vi "HumanExecute.vi"(8 "error in (no error)":errorcluster) -> (0 "error out":errorcluster)   [LabVIEW 2023]
doc: "Execute for Human\n\ninput:\n error in (cluster)\n\noutput:\n error out (cluster)"
uses:
  <vilib>/Rock Robotics/WPI/Joystick/XBox Axes Indexer.ctl
  <vilib>/Rock Robotics/WPI/Joystick/XBox Buttons Indexer.ctl
  <vilib>/Rock Robotics/WPI/ThirdParty/JAS_Junk/TrajLib/VI/DigSeqLogic_Edge_On.vi
  <vilib>/Rock Robotics/WPI/ThirdParty/JAS_Junk/TrajLib/MathUtil_ApplyDeadband.vi
  Intake/IntakeCancelSendCmd.vi
  Intake/IntakeAlgaeSendCmd.vi
  Intake/IntakeDepositAlgaeSendCmd.vi
  Intake/IntakeCoralSendCmd.vi
  Intake/IntakeDepositCoralSendCmd.vi
  Elevator/ElevatorBargeSendCmd.vi
  Elevator/ElevatorSourceSendCmd.vi
  Elevator/ElevatorFloorSendCmd.vi
  Elevator/ElevSendDecCmd.vi
  Elevator/ElevSendIncCmd.vi
  Elevator/ElevatorCancelCmd.vi
  Elevator/ElevatorL4SendCmd.vi
  Elevator/ElevatorAlgae1SendCmd.vi
  Elevator/ElevatorL3SendCmd.vi
  Elevator/ElevatorAlgae2SendCmd.vi
  Elevator/ElevatorL2SendCmd.vi
  Elevator/ElevatorRestSendCmd.vi
  Elevator/ElevatorL1SendCmd.vi
  HumanGlobal.vi
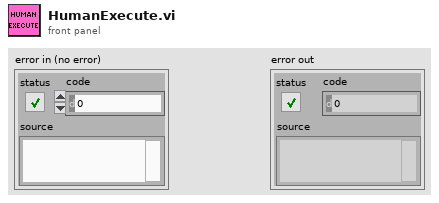
[diagram p1: front panel]
types:
  T1 = typedef "XBox Buttons Indexer.ctl" = enum16{"A", "B", "X", "Y", "Left Bumper", "Right Bumper", "Back", "Start", "Left Joystick", "Right Joystick"}
  T2 = typedef "XBox Axes Indexer.ctl" = enum16{"Left X", "Left Y", "Left Trigger", "Right Trigger", "Right X", "Right Y"}
  T3 = typedef "WPI_JoystickDevRef.ctl" = cluster{"Device":T4}
  T4 = typedef "WPI_JoystickDeviceEnum.ctl" = enum16{"USB 0", "USB 1", "USB 2", "USB 3", "USB 4", "USB 5"}
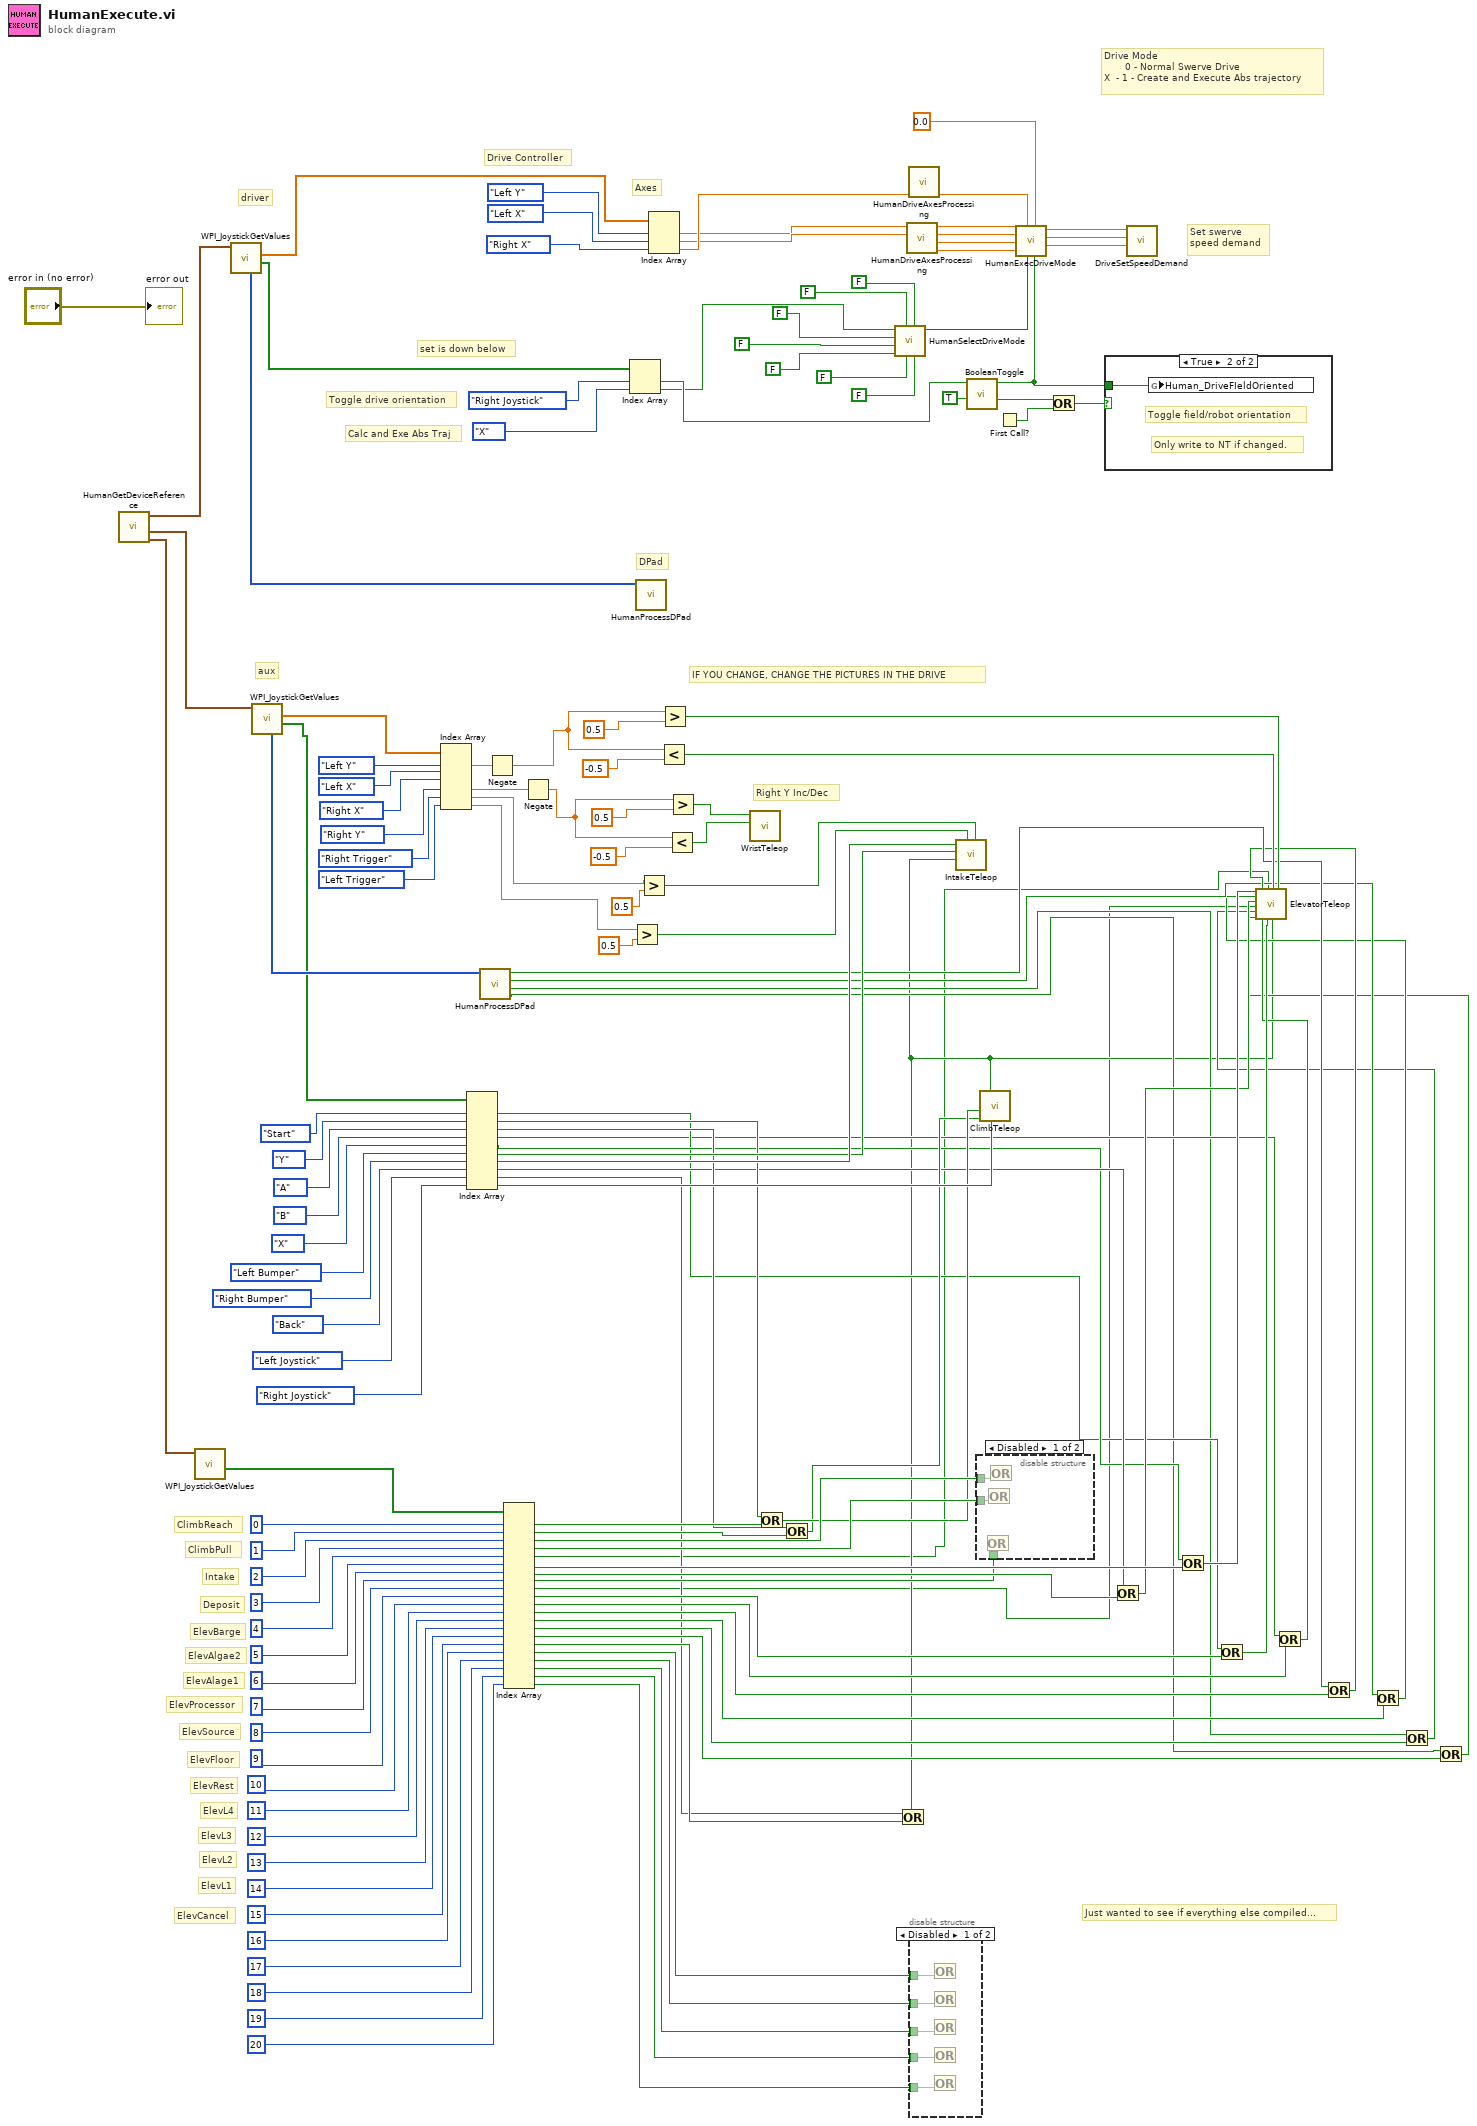
[diagram p0: block diagram]
diagram:
  # "ElevCancel"
  # "ElevL1"
  # "ElevL2"
  # "ElevL3"
  # "ElevL4"
  # "ElevRest"
  # "ElevFloor"
  # "ElevSource"
  # "ElevProcessor"
  # "ElevAlage1"
  # "ElevAlgae2"
  # "ElevBarge"
  # "Deposit"
  # "Intake"
  # "ClimbPull"
  # "ClimbReach"
  # "Just wanted to see if everything else compiled..."
  # "Right Y Inc/Dec"
  # "IF YOU CHANGE, CHANGE THE PICTURES IN THE DRIVE"
  # "DPad"
  # "Toggle drive orientation"
  # "Drive Mode\n       0 - Normal Swerve Drive\nX  - 1 - Create and Execute Abs trajectory"
  # "Calc and Exe Abs Traj"
  # "set is down below"
  # "Set swerve\nspeed demand"
  # "Axes"
  # "Drive Controller"
  # "aux"
  # "driver"
  n1 = call "HumanGetDeviceReference.vi"() -> ("AuxButtonBoard"=w66:T3, "Aux Joy"=w142:T3, "Driver Joy"=w143:T3)  [unwired: 8 in, 1 out]
  n2 = call <vilib>:"WPI_JoystickGetValues.vi"("JoystickDevRef"=w66) -> ("Buttons"=w65:bool[])  [unwired: 6 in, 4 out]
  n3 = call <vilib>:"WPI_JoystickGetValues.vi"("JoystickDevRef"=w143) -> ("Buttons"=w83:bool[], "Axes"=w138:dbl[], "POVs"=w110:i16[])  [unwired: 6 in, 2 out]
  n4 = call <vilib>:"WPI_JoystickGetValues.vi"("JoystickDevRef"=w142) -> ("Buttons"=w112:bool[], "Axes"=w111:dbl[], "POVs"=w113:i16[])  [unwired: 6 in, 2 out]
  n5 = Index Array(array=w111, index #1=XBox_Axes_Indexer."Left Y" ("XBox Axes"), index #2=XBox_Axes_Indexer."Left X" ("XBox Axes"), index #3=XBox_Axes_Indexer."Right X" ("XBox Axes"), index #4=XBox_Axes_Indexer."Right Y" ("XBox Axes"), index #5=XBox_Axes_Indexer."Right Trigger" ("XBox Axes"), index #6=XBox_Axes_Indexer."Left Trigger" ("XBox Axes")) -> (element #1=w70:dbl, element #4=w75:dbl, element #5=w102:dbl, element #6=w101:dbl)  [unwired: 2 out]
  n6 = Index Array "Index Array"(array=w112, index #1=XBox_Buttons_Indexer."Start" ("Nothing"), index #2=XBox_Buttons_Indexer."Y" ("OpenCloseClaw"), index #3=XBox_Buttons_Indexer."A" ("GrabberIn"), index #4=XBox_Buttons_Indexer."B" ("GrabberOut"), index #5=XBox_Buttons_Indexer."X" ("Nothing"), index #6=XBox_Buttons_Indexer."Left Bumper" ("Nothing"), index #7=XBox_Buttons_Indexer."Right Bumper" ("Nothing"), index #8=XBox_Buttons_Indexer."Back" ("Place Cone"), index #9=XBox_Buttons_Indexer."Left Joystick" ("Place Cone"), index #10=XBox_Buttons_Indexer."Right Joystick" ("Place Cone")) -> (element #1=w16:bool, element #2=w25:bool, element #3=w23:bool, element #4=w14:bool, element #5=w17:bool, element #6=w80:bool, element #7=w98:bool, element #8=w20:bool, element #9=w4:bool, element #10=w73:bool)
  n7 = call "HumanProcessDPad.vi"("POV"=w113) -> ("Left"=w6:bool, "Down"=w8:bool, "Right"=w10:bool, "Up"=w12:bool)  [unwired: 7 in]
  n8 = Negate(x=w70) -> (-x=w69:dbl)
  n9 = Index Array "Index Array"(array=w65, index #1=0 ("index"), index #2=1 ("index"), index #3=2 ("index"), index #4=3 ("index"), index #5=4 ("index"), index #6=5 ("index"), index #7=6 ("index"), index #8=7 ("index"), index #9=8 ("index"), index #10=9 ("index"), index #11=10 ("index"), index #12=11 ("index"), index #13=12 ("index"), index #14=13 ("index"), index #15=14 ("index"), index #16=15 ("index"), index #17=16 ("index"), index #18=17 ("index"), index #19=18 ("index"), index #20=19 ("index"), index #21=20 ("index")) -> (element #1=w43:bool, element #2=w42:bool, element #3=w41:bool, element #4=w40:bool, element #5=w2:bool, element #6=w39:bool, element #7=w38:bool, element #8=w18:bool, element #9=w1:bool, element #10=w37:bool, element #11=w36:bool, element #12=w35:bool, element #13=w34:bool, element #14=w33:bool, element #15=w32:bool, element #16=w31:bool, element #17=w30:bool, element #18=w29:bool, element #19=w28:bool, element #20=w27:bool, element #21=w26:bool)
  n10 = Negate(x=w75) -> (-x=w74:dbl)
  n11 = Index Array(array=w83, index #1=XBox_Buttons_Indexer."Right Joystick" ("Nothing"), index #2=XBox_Buttons_Indexer."X" ("Nothing")) -> (element #1=w81:bool, element #2=w77:bool)
  n12 = Greater?(x=w101, y=0.5) -> (0:w99:bool)
  n13 = call "HumanProcessDPad.vi"("POV"=w110) -> ()  [unwired: 7 in, 4 out]
  n14 = Greater?(x=w102, y=0.5) -> (0:w100:bool)
  n15 = Index Array(array=w138, index #1=XBox_Axes_Indexer."Left Y" ("XBox Axes"), index #2=XBox_Axes_Indexer."Left X" ("XBox Axes"), index #3=XBox_Axes_Indexer."Right X" ("XBox Axes")) -> (element #1=w127:dbl, element #2=w128:dbl, element #3=w129:dbl)
  n16 = Less?(x=w69, y=-0.5) -> (x < y?=w71:bool)
  n17 = Greater?(x=w69, y=0.5) -> (0:w72:bool)
  n18 = Less?(x=w74, y=-0.5) -> (x < y?=w67:bool)
  n19 = Greater?(x=w74, y=0.5) -> (0:w68:bool)
  n20 = call "WristTeleop.vi"("Dec"=w67, "Inc"=w68) -> ()  [unwired: 10 in]
  n21 = Or(x=w25, y=w43) -> (x .or. y?=w24:bool)
  n22 = Or(x=w23, y=w42) -> (x .or. y?=w22:bool)
  n23 = call "HumanSelectDriveMode.vi"("AutoTrajStageLeft"=FALSE, "AutoTrajSource"=FALSE, "AutoTrajStageCenter"=FALSE, "AutoTrajAmp"=FALSE, "AutoTrajSpeakerRight"=FALSE, "AutoTrajSpeakerCenter"=FALSE, "AutoTrajStageRight"=FALSE, "CalcAndExeAbsTraj"=w77) -> ("Drive Mode"=w97:i32)  [unwired: 3 in]
  n24 = Or(x=w4, y=w31) -> (x .or. y?=w3:bool)
  n25 = call "HumanDriveAxesProcessing.vi"("Left X"=w128, "Left Y"=w127) -> ("Right X"=w130:dbl, "Right Y"=w136:dbl, "Left X"=w137:dbl, "Left Y"=w135:dbl)  [unwired: 6 in]
  n26 = call "HumanDriveAxesProcessing.vi"("Right X"=w129) -> ("Right X"=w131:dbl)  [unwired: 7 in, 3 out]
  n27 = disable-structure shown="Disabled" {
    disable-tunnel: w30 -> [w149 _]
    disable-tunnel: w29 -> [w148 _]
    disable-tunnel: w28 -> [w147 _]
    disable-tunnel: w27 -> [w146 _]
    disable-tunnel: w26 -> [w145 _]
    frame Disabled {
      n28 = Or(y=w149) -> ()  [unwired: 1 in, 1 out]
      n29 = Or(y=w148) -> ()  [unwired: 1 in, 1 out]
      n30 = Or(y=w147) -> ()  [unwired: 1 in, 1 out]
      n31 = Or(y=w146) -> ()  [unwired: 1 in, 1 out]
      n32 = Or(y=w145) -> ()  [unwired: 1 in, 1 out]
    }
    frame Enabled {
    }
  }
  n33 = call "IntakeTeleop.vi"("CmdIntakeCoral"=w100, "CmdIntakeAlgae"=w99, "CmdIntakeCancel"=w3, "CmdIntakeDepositAlgae"=w80, "CmdIntakeDepositCoral"=w98) -> ()  [unwired: 7 in]
  n34 = call "BooleanToggle.vi"("InitialState"=TRUE, "Toggle Edge In"=w81) -> ("Changed"=w85:bool, "Output"=w84:bool)  [unwired: 8 in]
  n35 = disable-structure shown="Disabled" {
    disable-tunnel: w41 -> [w152 _]
    disable-tunnel: w40 -> [w151 _]
    disable-tunnel: w18 -> [w150 _]
    frame Disabled {
      n36 = Or(y=w150) -> ()  [unwired: 1 in, 1 out]
      n37 = Or(y=w151) -> ()  [unwired: 1 in, 1 out]
      n38 = Or(y=w152) -> ()  [unwired: 1 in, 1 out]
    }
    frame Enabled {
    }
  }
  n39 = call "ClimbTeleop.vi"("ClimbRest"=w73, "ClimbCancel"=w3, "ClimbPull"=w22, "ClimbReach"=w24) -> ()  [unwired: 8 in]
  n40 = First Call?() -> (First Call?: T/F=w87:bool)
  n41 = call "HumanExecDriveMode.vi"("Enable Field Oriented Drive"=w84, "AutoSpeakerAngle"=0.0, "State"=w97, "Rotation"=w131, "Right X"=w130, "Right Y"=w136, "Left X"=w137, "Left Y"=w135) -> ("AMotorDemand"=w134:dbl, "YMotorDemand"=w133:dbl, "XMotorDemand"=w132:dbl)  [unwired: 1 in]
  n42 = Or(x=w85, y=w87) -> (x .or. y?=w88:bool)
  n43 = case shown="True" w88 {
    tunnel: w84 -> [_ w153]
    frame False {
    }
    frame True {
      # "Only write to NT if changed."
      # "Toggle field/robot orientation"
      n44 = global write "HumanGlobal.vi" "Human_DriveFIeldOriented"(w153) -> ()
    }
  }
  n45 = Or(x=w20, y=w38) -> (x .or. y?=w19:bool)
  n46 = call "DriveSetSpeedDemand.vi"("ASpeedDemand (d/s)"=w134, "YSpeedDemand (ft/s)"=w133, "XSpeedDemand (ft/s)"=w132) -> ()  [unwired: 9 in]
  n47 = Or(x=w17, y=w39) -> (x .or. y?=w21:bool)
  n48 = Or(x=w16, y=w37) -> (x .or. y?=w15:bool)
  n49 = Or(x=w14, y=w36) -> (x .or. y?=w13:bool)
  n50 = Or(x=w12, y=w35) -> (x .or. y?=w11:bool)
  n51 = Or(x=w10, y=w34) -> (x .or. y?=w9:bool)
  n52 = Or(x=w8, y=w33) -> (x .or. y?=w7:bool)
  n53 = Or(x=w6, y=w32) -> (x .or. y?=w5:bool)
  n54 = call "ElevatorTeleop.vi"("CmdElevAlgae2"=w21, "CmdElevL3"=w9, "CmdElevAlgae1"=w19, "CmdElevSource"=w1, "CmdElevL2"=w7, "CmdElevL1"=w5, "CmdElevL4"=w11, "CmdElevRest"=w13, "CmdBarge"=w2, "CmdFloor"=w15, "CmdElevDec"=w71, "CmdElevCancel"=w3, "CmdElevInc"=w72) -> ()  [unwired: 7 in]
  "error out" <- "error in (no error)"
